vi "set tcp ip server ref id.vi"(8 "error in (no error)":errorcluster, 9 "Connected?":bool, 10 "tcp ID":refnum<k5>, 11 "tcp ip server in":refnum<class "tcp ip server.lvclass">) -> (0 "error out":errorcluster, 3 "tcp ip server out":refnum<class "tcp ip server.lvclass">)   [LabVIEW 2020, in "tcp ip server.lvclass"]
uses:
  tcp ip server.lvclass
  tcp ip server.lvclass/tcp ip server.ctl
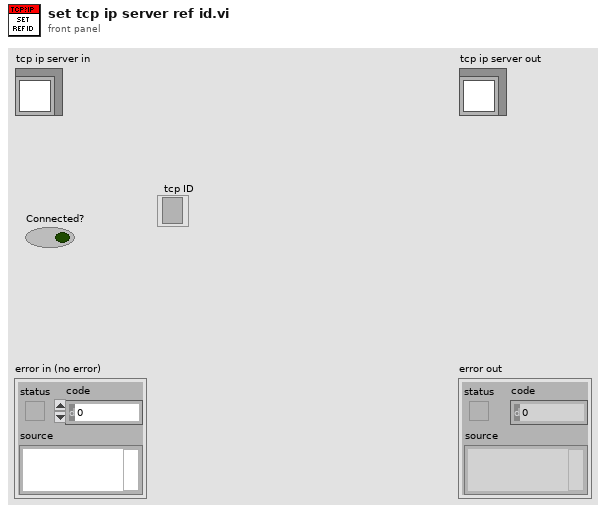
[diagram p1: front panel]
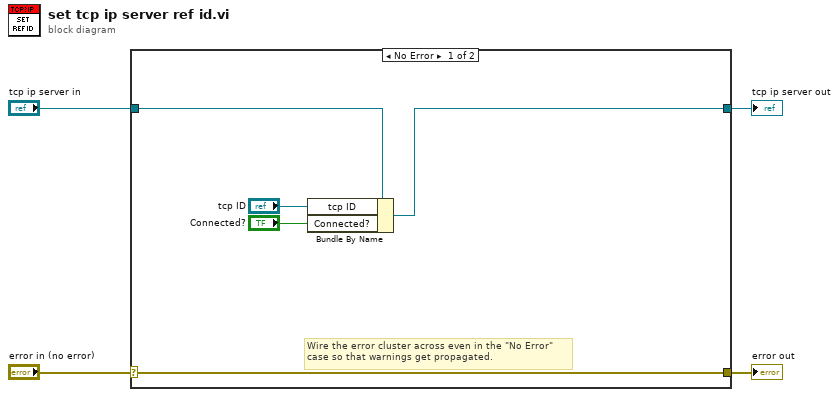
[diagram p0: block diagram]
diagram:
  n1 = case shown="No Error" "error in (no error)" {
    selector: "error in (no error)" -> [w9 w11]
    tunnel: [w9 w11] -> w3
    tunnel: [w6 w10] -> w1
    tunnel: "tcp ip server in" -> [w7 w10]
    frame No Error {
      # "Wire the error cluster across even in the \"No Error\"\ncase so that warnings get propagated."
      n2 = Bundle By Name(cluster=w7, "tcp ID"="tcp ID", "Connected?"="Connected?") -> (w6:refnum<class "tcp ip server.lvclass">)
    }
    frame Error {
    }
  }
  "error out" <- w3
  "tcp ip server out" <- w1
